vi "Cargar MXN.vi"(7 "MXN Actor.lvlib:MXN Actor.lvclass":refnum<class "MXN Actor.lvclass">) -> (5 "MXN Actor.lvlib:MXN Actor.lvclass 2":refnum<class "MXN Actor.lvclass">)   [LabVIEW 2019, in "MXN Actor.lvlib" / "MXN Actor.lvclass"]
uses:
  MXN Actor.lvclass
  MXN Actor.lvclass/MXN Actor.ctl
  <vilib>/Utility/config.llb/Read Key (String).vi
  <vilib>/Utility/config.llb/NI_LVConfig.lvlib
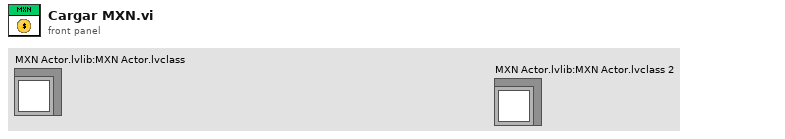
[diagram p1: front panel]
types:
  T1 = typedef "NI_LVConfig.lvlib/Config Data RefNum.ctl" = refnum<k1>
  T2 = cluster{"[0]":string, "[1]":string, "[2]":string, "[3]":string, "[4]":string, "[5]":string, "[6]":string, "[7]":string, "[8]":string}
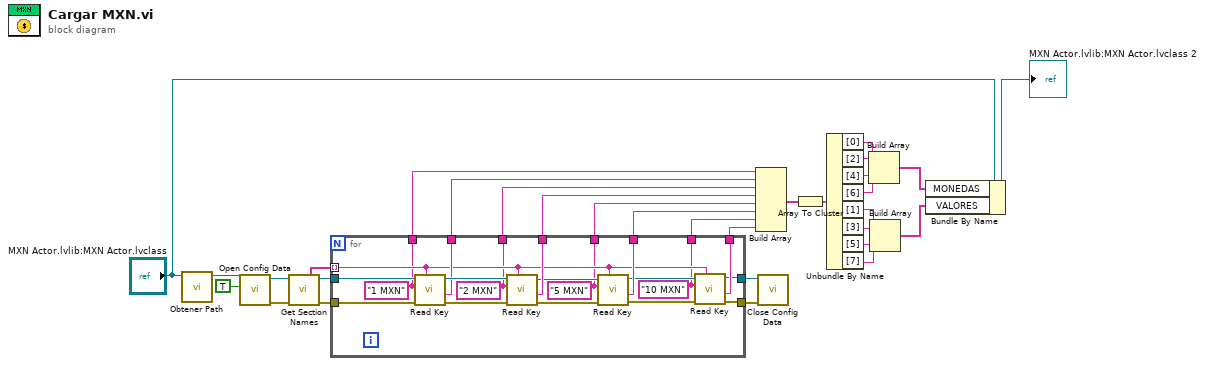
[diagram p0: block diagram]
diagram:
  n1 = call "Obtener Path.vi"("MXN Actor.lvlib:MXN Actor.lvclass"="MXN Actor.lvlib:MXN Actor.lvclass") -> ("appended path"=w23:path)  [unwired: 10 in]
  n2 = call <vilib>:"Open Config Data.vi"("create file if necessary (T)"=TRUE, "configuration file path"=w23) -> ("error out"=w30:errorcluster, "refnum"=w29:T1)  [unwired: 7 in, 1 out]
  n3 = call <vilib>:"Get Section Names.vi"("error in (no error)"=w30, "refnum"=w29) -> ("error out"=w27:errorcluster, "section names"=w24:string[], "refnum out"=w28:T1)  [unwired: 7 in]
  n4 = for {
    tunnel: w28 -> [w50]
    tunnel: w27 -> [w49]
    tunnel: w24 -> [w36] mode=indexing
    tunnel: [w40] -> w26
    tunnel: [w41] -> w25
    tunnel: [w47] -> w21
    tunnel: [w46] -> w19
    tunnel: [w45] -> w17
    tunnel: [w44] -> w15
    tunnel: [w35] -> w22
    tunnel: [w34] -> w20
    tunnel: [w33] -> w18
    tunnel: [w32] -> w16
    w32 = "10 MXN" ("key")
    w33 = "5 MXN" ("key")
    w34 = "2 MXN" ("key")
    w35 = "1 MXN" ("key")
    n5 = call-poly <vilib>:"Read Key.vi"("section"=w36, "error in (no error)"=w49, "key"=w35, "refnum"=w50) -> ("error out"=w37:errorcluster, "value"=w47:string, "refnum out"=w48:T1)  [unwired: 4 in, 1 out]
    n6 = call-poly <vilib>:"Read Key.vi"("section"=w36, "error in (no error)"=w37, "key"=w34, "refnum"=w48) -> ("error out"=w38:errorcluster, "value"=w46:string, "refnum out"=w42:T1)  [unwired: 4 in, 1 out]
    n7 = call-poly <vilib>:"Read Key.vi"("section"=w36, "error in (no error)"=w38, "key"=w33, "refnum"=w42) -> ("error out"=w39:errorcluster, "value"=w45:string, "refnum out"=w43:T1)  [unwired: 4 in, 1 out]
    n8 = call-poly <vilib>:"Read Key.vi"("section"=w36, "error in (no error)"=w39, "key"=w32, "refnum"=w43) -> ("error out"=w40:errorcluster, "value"=w44:string, "refnum out"=w41:T1)  [unwired: 4 in, 1 out]
  }
  n9 = Build Array(w22, w21, w20, w19, w18, w17, w16, w15) -> (w12:string[])
  n10 = call <vilib>:"Close Config Data.vi"("error in (no error)"=w26, "refnum"=w25) -> ()  [unwired: 8 in, 2 out]
  n11 = Array To Cluster(array=w12) -> (cluster=w11:T2)
  n12 = Unbundle By Name(w11) -> ("[0]"=w7:string, "[2]"=w10:string, "[4]"=w8:string, "[6]"=w9:string, "[1]"=w6:string, "[3]"=w5:string, "[5]"=w4:string, "[7]"=w3:string)
  n13 = Build Array(w7, w10, w8, w9) -> (w1:string[])
  n14 = Build Array(w6, w5, w4, w3) -> (w2:string[])
  n15 = Bundle By Name(cluster="MXN Actor.lvlib:MXN Actor.lvclass", "MONEDAS"=w1, "VALORES"=w2) -> (→"MXN Actor.lvlib:MXN Actor.lvclass 2":refnum<class "MXN Actor.lvclass">)
